vi "Remove uneeded lines.vi"(11 "Array":string[](array[string])) -> (3 "Array out":string[](array[string]))   [LabVIEW 2013]
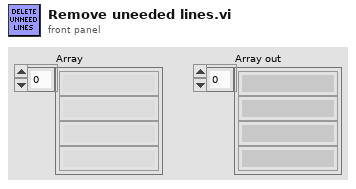
[diagram p1: front panel]
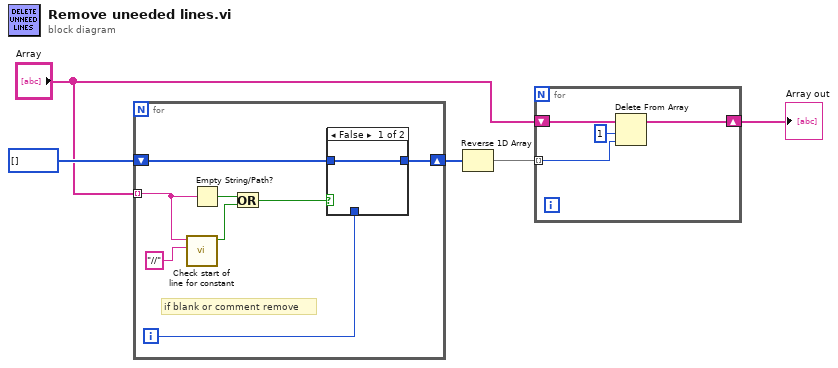
[diagram p0: block diagram]
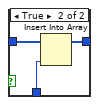
[diagram p2: hidden frame]
diagram:
  n1 = for {
    tunnel: "Array" -> [w12] mode=indexing
    shift-right: [w7] -> w4
    shift-left: i32[] [] -> [w6]
    i -> [w8]
    # "if blank or comment remove"
    n2 = call "Check start of line for constant.vi"("Constant to check start of line"="//", "Line"=w12) -> ("Does it start with constant?"=w11:bool)  [unwired: 9 in]
    n3 = Empty String/Path?(string/path=w12) -> (empty?=w10:bool)
    n4 = Or(x=w10, y=w11) -> (x .or. y?=w9:bool)
    n5 = case shown="False" w9 {
      tunnel: w8 -> [_ w17]
      tunnel: [w14 w15] -> w7
      tunnel: w6 -> [w14 w16]
      frame False {
      }
      frame True {
        n6 = Insert Into Array(array=w16, new element=w17) -> (w15:i32[])  [unwired: 1 in]
      }
    }
  }
  n7 = Reverse 1D Array(array=w4) -> (reversed array=w3:i32[])
  n8 = for {
    tunnel: w3 -> [w20] mode=indexing
    shift-right: [w18] -> w1
    shift-left: "Array" -> [w21]
    n9 = Delete From Array(array=w21, length=1, index=w20) -> (array with subset deleted=w18:string[])  [unwired: 1 out]
  }
  "Array out" <- w1
